vi "DataPacker_SendDataToMIDAS.vi"(0 "DataPacker in":refnum<class "DataPacker.lvclass">, 5 "data in":string, 9 "data in length":u32, 11 "error in (no error)":errorcluster) -> (4 "DataPacker out":refnum<class "DataPacker.lvclass">, 6 "MIDAS Reply":string, 8 "Send Time, Recieve Time":dbl[](array[numeric]), 10 "MIDAS Comm finished":timestamp, 15 "error out":errorcluster)   [LabVIEW 2018, in "feGEM DataPacker.lvlib" / "DataPacker.lvclass"]
uses:
  DataPacker.lvclass
  DataPacker.lvclass/DataPacker.ctl
  feGEM DataPacker.lvlib
panel:
  out "MIDAS Address":string
  out "bytes written":i32
  out "Port Number":u16
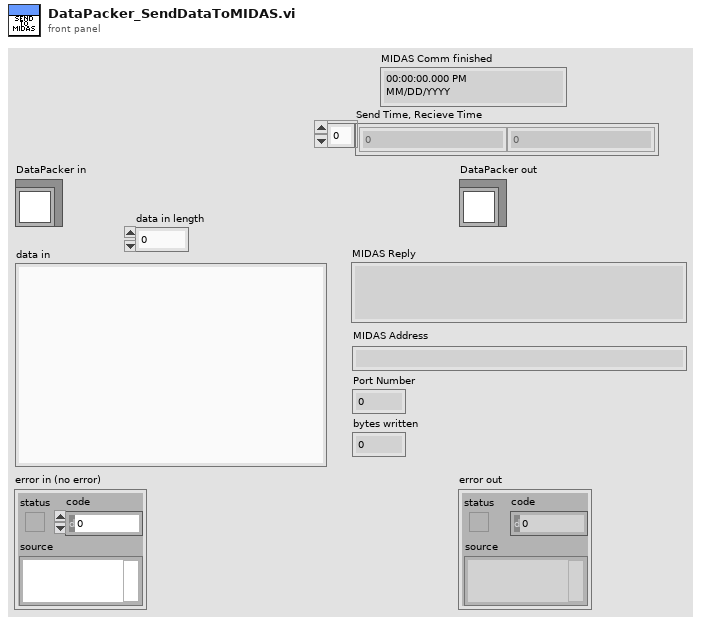
[diagram p1: front panel]
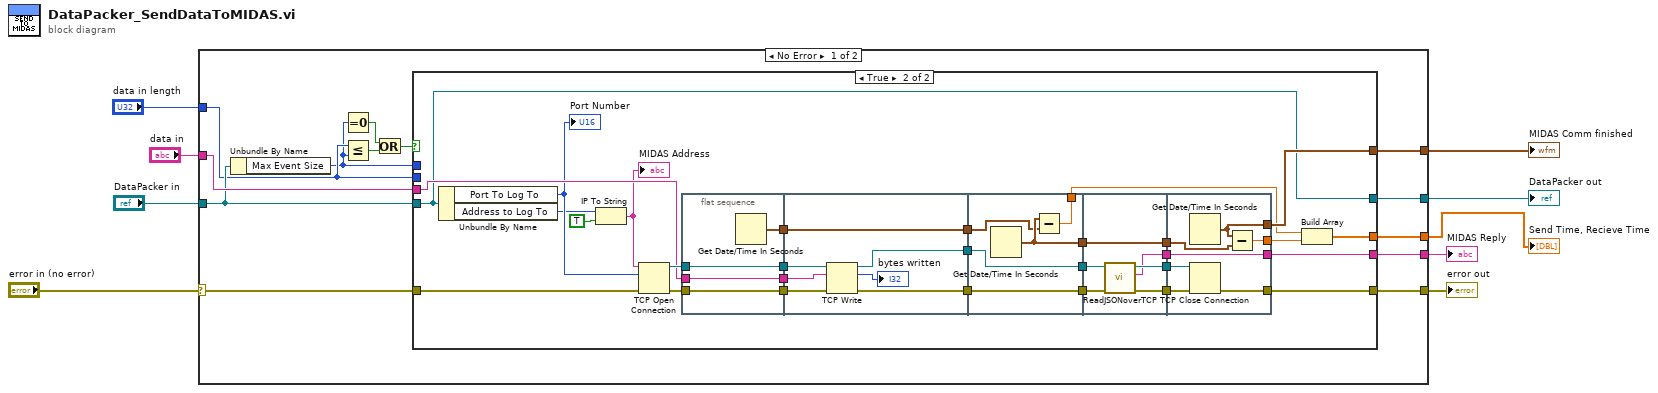
[diagram p0: block diagram]
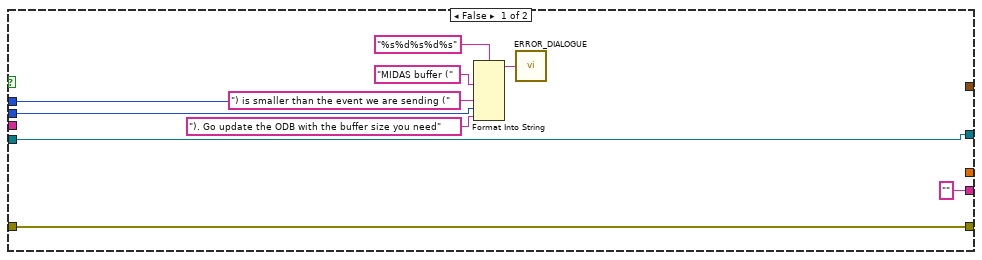
[diagram p2: hidden frame]
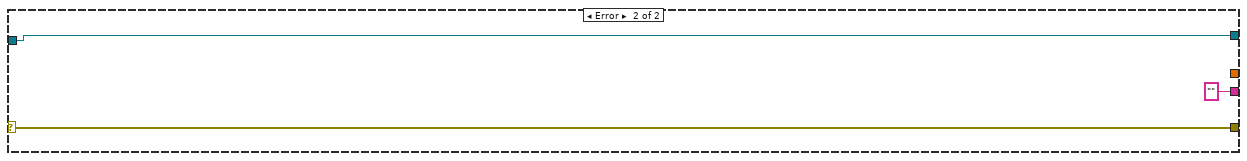
[diagram p3: hidden frame]
diagram:
  n1 = case shown="No Error" "error in (no error)" {
    selector: "error in (no error)" -> [w20 w93]
    tunnel: [w19 w93] -> w8
    tunnel: [w18 w92] -> w6
    tunnel: "DataPacker in" -> [w17 w92]
    tunnel: "data in" -> [w22 _]
    tunnel: [w21 ""] -> w4
    tunnel: "data in length" -> [w16 _]
    tunnel: [w11 _] -> w2
    tunnel: [w10 _] -> w1
    frame No Error {
      n2 = Unbundle By Name(w17) -> ("Max Event Size"=w15:u32)
      n3 = Equal To 0?(x=w15) -> (x = 0?=w14:bool)
      n4 = Less Or Equal?(x=w16, y=w15) -> (x <= y?=w13:bool)
      n5 = Or(x=w14, y=w13) -> (x .or. y?=w12:bool)
      n6 = case shown="True" w12 {
        tunnel: w22 -> [_ w59]
        tunnel: ["" w55] -> w21
        tunnel: w17 -> [w25 w37]
        tunnel: w20 -> [w24 w36]
        tunnel: [w24 w38] -> w19
        tunnel: [w25 w37] -> w18
        tunnel: w16 -> [w27 _]
        tunnel: w15 -> [w26 _]
        tunnel: [_ w47] -> w11
        tunnel: [_ w39] -> w10
        frame False {
          n7 = Format Into String(format string="%s%d%s%d%s", "MIDAS buffer (" ("input 1"), w26, ") is smaller than the event we are sending (" ("input 3"), w27, "). Go update the ODB with the buffer size you need" ("input 5")) -> (resulting string=w28:string)  [unwired: 2 in, 1 out]
          n8 = call "ERROR_DIALOGUE.vi"("String"=w28) -> ()
        }
        frame True {
          n9 = Unbundle By Name(w37) -> ("Port To Log To"=w58:u16, "Address to Log To"=w35:u32)
          "Port Number" <- w58
          n10 = IP To String(1:TRUE ("dot notation? (F)"), 2:w35) -> (0:w33:string)
          "MIDAS Address" <- w33
          n11 = TCP Open Connection(address=w33, remote port or service name=w58, error in (no error)=w36) -> (connection ID=w60:refnum<k5>, error out=w61:errorcluster)  [unwired: 2 in]
          n12 = flat-sequence {
            tunnel: w59 -> [w63]
            tunnel: w60 -> [w64]
            tunnel: w61 -> [w65]
            tunnel: [w65] -> w45
            tunnel: [w64] -> w44
            tunnel: [w63] -> w43
            tunnel: [w62] -> w42
            tunnel: [w71] -> w57
            tunnel: [w67] -> w54
            tunnel: [w66] -> w52
            tunnel: w45 -> [w72]
            tunnel: w44 -> [w70]
            tunnel: w43 -> [w69]
            tunnel: w42 -> [w66]
            tunnel: w57 -> [w77]
            tunnel: [w77] -> w56
            tunnel: w54 -> [w76]
            tunnel: [w76] -> w53
            tunnel: w52 -> [w74]
            tunnel: [w75] -> w51
            tunnel: [w73] -> w41
            tunnel: w56 -> [w81]
            tunnel: w53 -> [w82]
            tunnel: w51 -> [w83]
            tunnel: [w80] -> w50
            tunnel: [w78] -> w49
            tunnel: [w79] -> w48
            tunnel: [w83] -> w46
            tunnel: [w90] -> w55
            tunnel: w50 -> [w85]
            tunnel: w49 -> [w86]
            tunnel: w48 -> [w90]
            tunnel: [w89] -> w47
            tunnel: w46 -> [w88]
            tunnel: [w87] -> w40
            tunnel: [w84] -> w38
            frame #0 {
              n13 = Get Date/Time In Seconds() -> (seconds since 1Jan1904=w62:timestamp)
            }
            frame #1 {
              n14 = TCP Write(connection ID=w70, data in=w69, error in (no error)=w72) -> (connection ID out=w67:refnum<k5>, bytes written=→"bytes written":i32, error out=w71:errorcluster)  [unwired: 1 in]
            }
            frame #2 {
              n15 = Get Date/Time In Seconds() -> (seconds since 1Jan1904=w75:timestamp)
              n16 = Subtract(x=w75, y=w74) -> (x-y=w73:dbl)
            }
            frame #3 {
              n17 = call "ReadJSONoverTCP.vi"("error out"=w81, "connection ID"=w82) -> ("error out"=w78:errorcluster, "JSON"=w79:string, "connection ID"=w80:refnum<k5>)  [unwired: 7 in]
            }
            frame #4 {
              n18 = Get Date/Time In Seconds() -> (seconds since 1Jan1904=w89:timestamp)
              n19 = TCP Close Connection(connection ID=w85, error in (no error)=w86) -> (error out=w84:errorcluster)  [unwired: 1 in, 1 out]
              n20 = Subtract(x=w89, y=w88) -> (x-y=w87:dbl)
            }
          }
          n21 = Build Array(w41, w40) -> (w39:dbl[])
        }
      }
    }
    frame Error {
    }
  }
  "error out" <- w8
  "DataPacker out" <- w6
  "MIDAS Reply" <- w4
  "MIDAS Comm finished" <- w2
  "Send Time, Recieve Time" <- w1
